vi "ConfigureMarker.vi"(6 "Meas Name":string="MY_MEAS", 8 "error in (no error)":errorcluster, 9 "Marker":u32=1, 10 "Channel":u32=1, 11 "NetA_AgNA in":refnum<class "NetA_AgNA.lvclass">) -> (0 "error out":errorcluster, 3 "NetA_AgNA out":refnum<class "NetA_AgNA.lvclass">)   [LabVIEW 2014, in "NetA_AgNA.lvclass"]
doc: "Configures a marker associated with the specified measurement."
uses:
  NetA_AgNA.lvclass
  NetA_AgNA.lvclass/NetA_AgNA.ctl
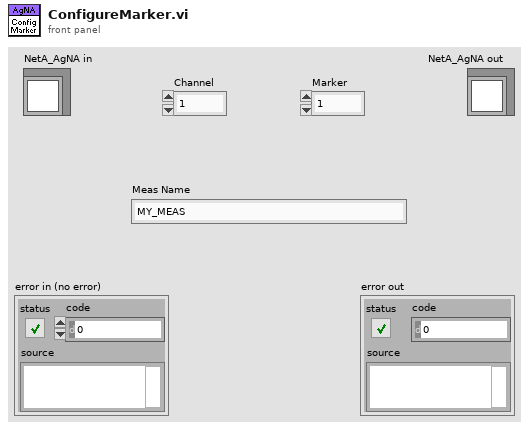
[diagram p1: front panel]
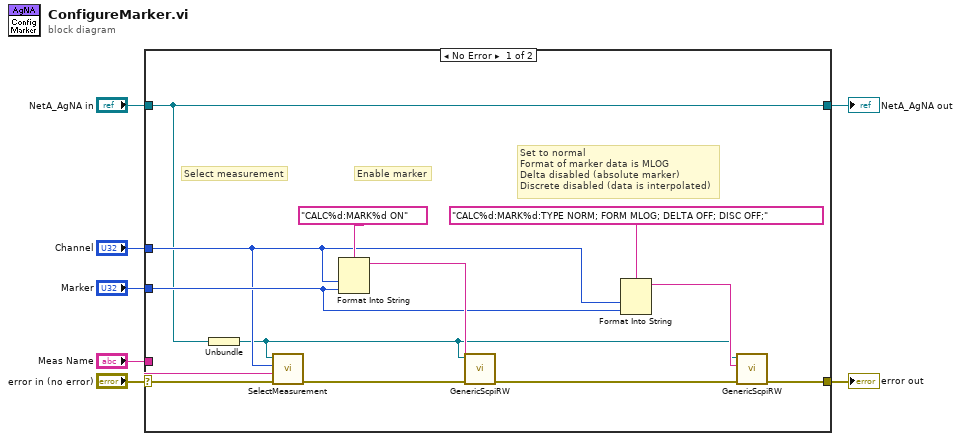
[diagram p0: block diagram]
diagram:
  n1 = case shown="No Error" "error in (no error)" {
    selector: "error in (no error)" -> [w14 w21]
    tunnel: "Marker" -> [w15 _]
    tunnel: "Channel" -> [w12 _]
    tunnel: "Meas Name" -> [w11 _]
    tunnel: "NetA_AgNA in" -> [w9 w22]
    tunnel: [w9 w22] -> w2
    tunnel: [w10 w21] -> w1
    frame No Error {
      # "Select measurement"
      # "Set to normal\nFormat of marker data is MLOG\nDelta disabled (absolute marker)\nDiscrete disabled (data is interpolated)"
      # "Enable marker"
      n2 = Unbundle(w9) -> (w8:refnum<k15>)
      n3 = call "SelectMeasurement.vi"("error in (no error)"=w14, "Meas Name"=w11, "Channel"=w12, "resource name"=w8) -> ("error out"=w13:errorcluster)  [unwired: 7 in]
      n4 = Format Into String(format string="CALC%d:MARK%d ON", w12, w15) -> (resulting string=w18:string)  [unwired: 2 in, 1 out]
      n5 = call "GenericScpiRW.vi"("error in (no error)"=w13, "SCPI Command"=w18, "resource name"=w8) -> ("error out"=w20:errorcluster)  [unwired: 7 in, 1 out]
      n6 = Format Into String(format string="CALC%d:MARK%d:TYPE NORM; FORM MLOG; DELTA OFF; DISC OFF;" ("ChannelType"), w12, w15) -> (resulting string=w17:string)  [unwired: 2 in, 1 out]
      n7 = call "GenericScpiRW.vi"("error in (no error)"=w20, "SCPI Command"=w17, "resource name"=w8) -> ("error out"=w10:errorcluster)  [unwired: 7 in, 1 out]
    }
    frame Error {
    }
  }
  "error out" <- w1
  "NetA_AgNA out" <- w2
